vi "SubPanel_Import Export Value.vi"(4 "SubPanel Function Select":T1, 5 "Sub Panel":refnum<vi>, 6 "Border Spacing":i32=-2, 7 "VI":refnum<vi>, 8 "Error":errorcluster, 9 "Frame Ref":refnum<vi>, 10 "Ctl Refnum":refnum<vi>, 11 "Value":variant) -> (0 "Error Out":errorcluster, 3 "Value Out":variant)   [LabVIEW 2015]
uses:
  TypeDefs_Utility/ENUM_SubPanel_Select.ctl
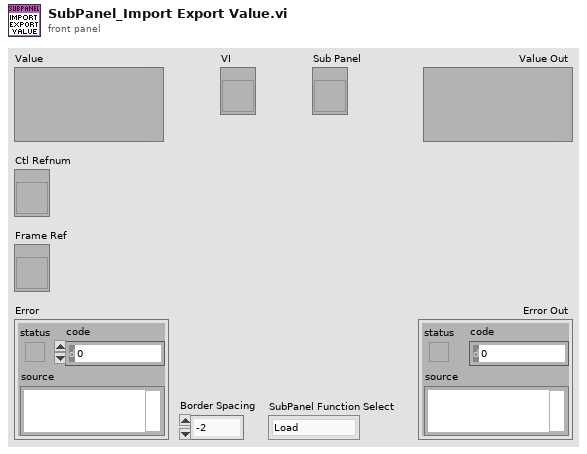
[diagram p1: front panel]
types:
  T1 = typedef "ENUM_SubPanel_Select.ctl" = enum16{"Load", "Data to Display", "Display to Data", "Unload"}
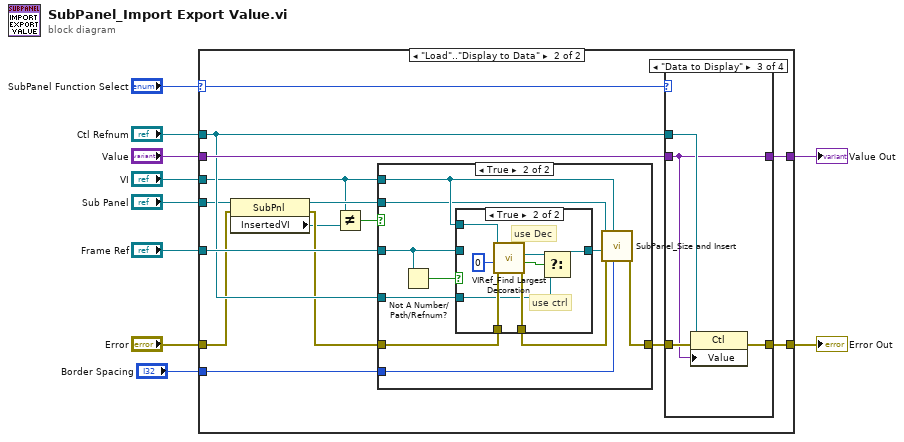
[diagram p0: block diagram]
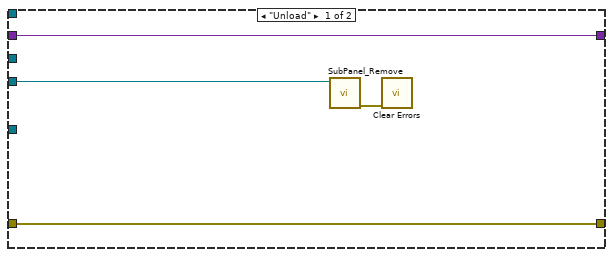
[diagram p2: hidden frame]
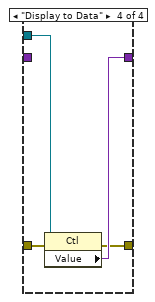
[diagram p7: hidden frame]
diagram:
  n1 = case shown="\"Load\"..\"Display to Data\"" "SubPanel Function Select" {
    selector: "SubPanel Function Select" -> [_ w22]
    tunnel: "Value" -> [w12 w29]
    tunnel: [w12 w28] -> w9
    tunnel: [w13 w27] -> w8
    tunnel: "Sub Panel" -> [w14 w21]
    tunnel: "Border Spacing" -> [_ w25]
    tunnel: "Frame Ref" -> [_ w24]
    tunnel: "VI" -> [_ w17]
    tunnel: "Ctl Refnum" -> [_ w23]
    tunnel: "Error" -> [w13 w20]
    frame "Unload" {
      n2 = call "SubPanel_Remove.vi"("SubPanel"=w14) -> ("Error Out"=w11:errorcluster)  [unwired: 9 in, 1 out]
      n3 = call <vilib>:"Clear Errors.vi"("error in (no error)"=w11) -> ()  [unwired: 5 in, 2 out]
    }
    frame "Load".."Display to Data" {
      n4 = property class="SubPnl"(reference=w21, error in=w20) -> (reference out=w18:refnum<vi>, error out=w19:errorcluster, "InsertedVI"=w16:refnum<vi>)
      n5 = Not Equal?(x=w17, y=w16) -> (x != y?=w15:bool)
      n6 = case shown="True" w15 {
        tunnel: [w30 w40] -> w26
        tunnel: w25 -> [_ w39]
        tunnel: w24 -> [_ w37]
        tunnel: w17 -> [_ w35]
        tunnel: w23 -> [_ w34]
        tunnel: w18 -> [_ w32]
        tunnel: w19 -> [w30 w31]
        frame False {
        }
        frame True {
          n7 = Not A Number/Path/Refnum?(number/path/refnum=w37) -> (NaN/Path/Refnum?=w38:bool)
          n8 = case shown="True" w38 {
            tunnel: w37 -> [w42 _]
            tunnel: [w42 w44] -> w36
            tunnel: w35 -> [_ w50]
            tunnel: w34 -> [_ w43]
            tunnel: w31 -> [w41 w48]
            tunnel: [w41 w47] -> w33
            frame False {
              # "Use Frame"
            }
            frame True {
              # "use Dec"
              # "use ctrl"
              n9 = call "VIRef_Find Largest Decoration.vi"("Error"=w48, "Decoration index"=0, "VI's Ref"=w50) -> ("Error Out"=w47:errorcluster, "Found"=w46:bool, "Decor Refnum Out"=w45:refnum<vi>)  [unwired: 2 in, 4 out]
              n10 = Select(t=w45, s=w46, f=w43) -> (s? t:f=w44:refnum<vi>)
            }
          }
          n11 = call "SubPanel_Size and Insert.vi"("Border Spacing"=w39, "VI"=w35, "Error"=w33, "Frame Ref"=w36, "Sub Panel"=w32) -> ("Error Out"=w40:errorcluster)  [unwired: 3 in, 3 out]
        }
      }
      n12 = case shown="\"Data to Display\"" w22 {
        tunnel: w26 -> [w51 w54 w57 w60]
        tunnel: [w51 w54 w56 w59] -> w27
        tunnel: w23 -> [_ _ w58 w62]
        tunnel: [w52 w53 w55 w61] -> w28
        tunnel: w29 -> [w52 w53 w55 _]
        frame "Unload" {
        }
        frame "Load" {
        }
        frame "Data to Display" {
          n13 = property class="Ctl"(reference=w58, error in=w57, "Value"=w55) -> (error out=w56:errorcluster)  [unwired: 1 out]
        }
        frame "Display to Data" {
          n14 = property class="Ctl"(reference=w62, error in=w60) -> (error out=w59:errorcluster, "Value"=w61:variant)  [unwired: 1 out]
        }
      }
    }
  }
  "Value Out" <- w9
  "Error Out" <- w8
